vi "vPR_All.vi"(8 "error in (no error)":errorcluster, 9 "結束時間":timestamp=timestamp(3738902301.8455286 s since 1904-01-01), 10 "開始時間":timestamp=timestamp(3738815886.436984 s since 1904-01-01), 11 "DBlink":string="Driver={ODBC Driver 17 for SQL Server};Server=localhost\\SQLEXPRESS;Database=ZDX201;UID=labview;PWD=Dsa@54137926") -> (0 "error out":errorcluster={"status"=TRUE, "code"=-2147217843, "source"="NI_Database_API.lvlib:DB Tools Open Connec (String).vi->WD_assemble_data.vi<ERR>ADO Error: 0x80040E4D\r\nException occured in Microsoft OLE DB Provider for ODBC Drivers: [Microsoft][ODBC Driver 17 for SQL Server][SQL Server]使用者 'labview' 的登入失敗。 in NI_Database_API.lvlib:DB Tools Open Connec (String).vi->WD_assemble_data.vi"}, 3 "Production":T1(array[cluster]))   [LabVIEW 2019]
uses:
  <vilib>/addons/database/Connection.llb/DB Tools Open Connec (String).vi
  <vilib>/addons/database/Connection.llb/Conn Execute.vi
  <vilib>/addons/database/Recordset.llb/Rec Fetch Recordset Data (R).vi
  <vilib>/addons/database/Recordset.llb/Rec Destroy - Connection.vi
  <vilib>/addons/database/_DB Variant To Data/Database Variant To Data.xnode
  <vilib>/addons/database/NI_Database_API.lvlib
panel:
  out "查詢結果":string="SELECT [id]\n      ,[name]\n      ,[barcode A]\n      ,[barcode B]\n      ,[update_time]\n  FROM [ZDX201].[dbo].[workplace_data]\n  where id>0 and id<6\n  order by id"
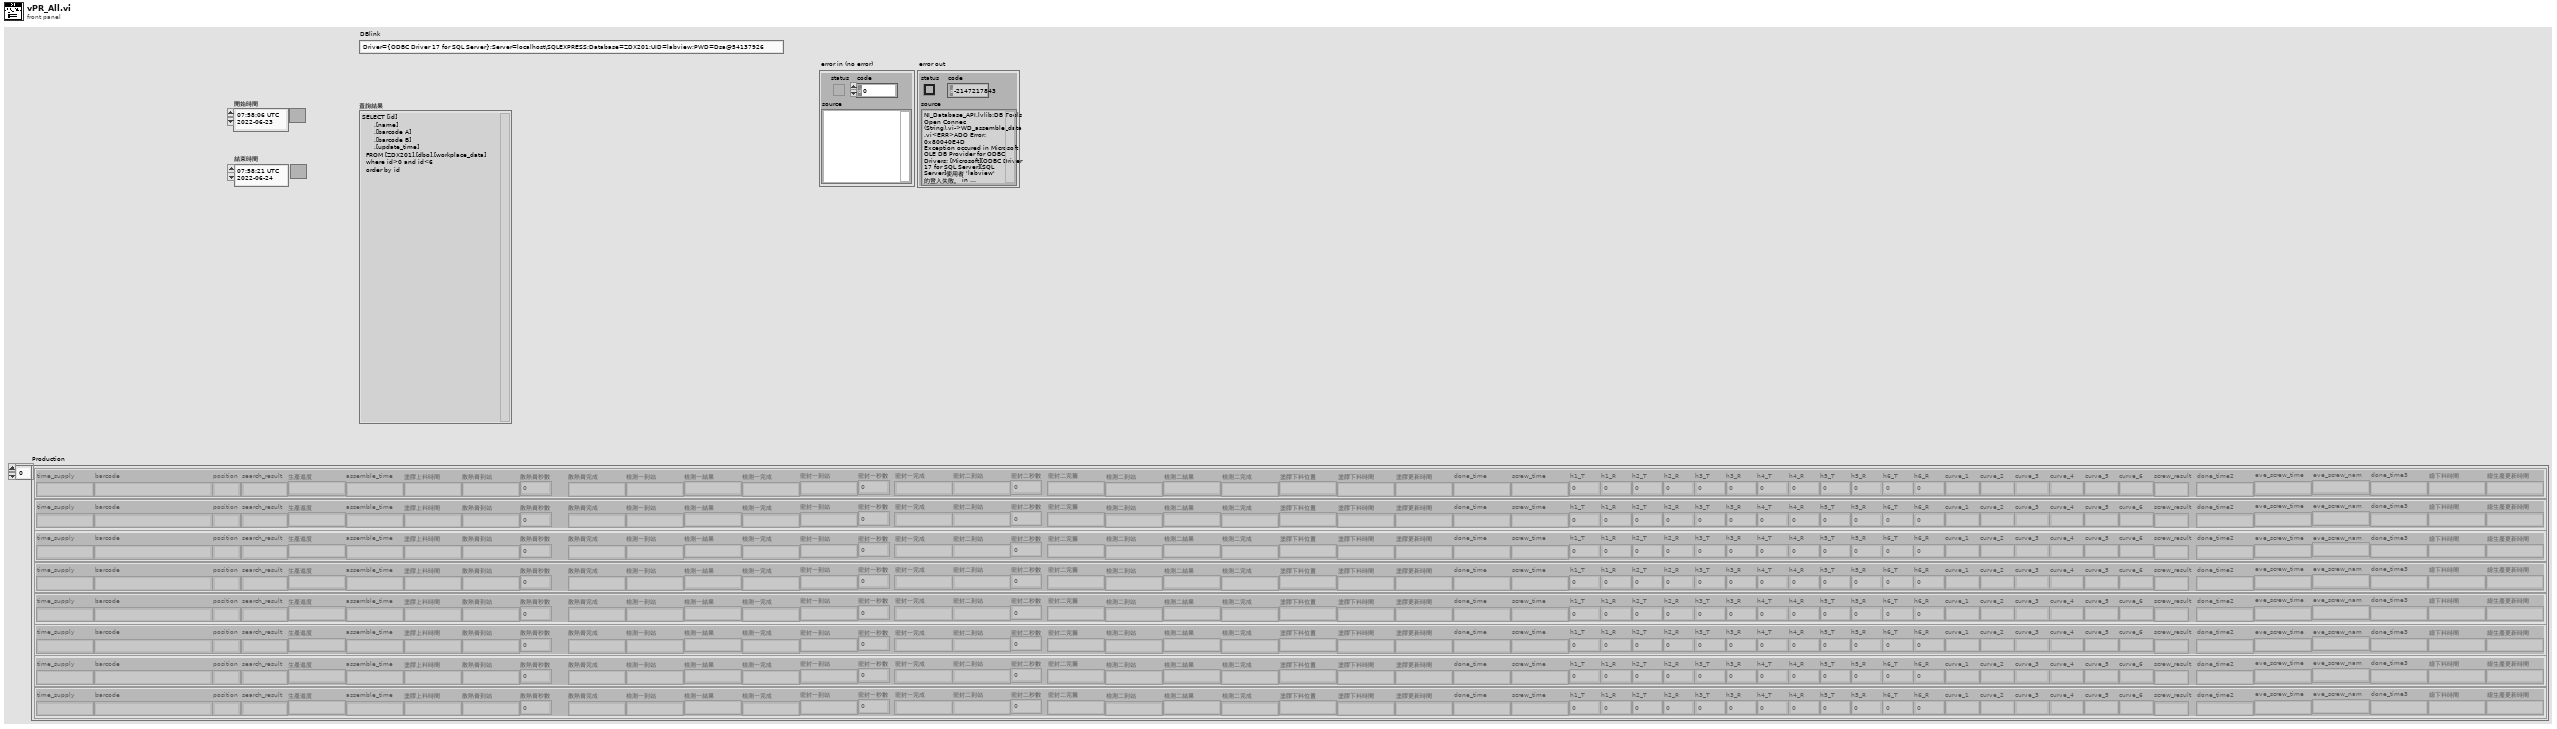
[diagram p1: front panel]
types:
  T1 = cluster{"time_supply":string, "barcode":string, "position":string, "search_result":string, "生產進度":string, "assemble_time":string, "塗膠上料時間":string, "散熱膏到站":string, "散熱膏秒數":dbl, "散熱膏完成":string, "檢測一到站":string, "檢測一結果":string, "檢測一完成":string, "密封一到站":string, "密封一秒數":dbl, "密封一完成":string, "密封二到站":string, "密封二秒數":dbl, "密封二完籌":string, "檢測二到站":string, "檢測二結果":string, "檢測二完成":string, "塗膠下料位置":string, "塗膠下料時間":string, "塗膠更新時間":string, "done_time":string, "screw_time":string, "h1_T":dbl, "h1_R":dbl, "h2_T":dbl, "h2_R":dbl, "h3_T":dbl, "h3_R":dbl, "h4_T":dbl, "h4_R":dbl, "h5_T":dbl, "h5_R":dbl, "h6_T":dbl, "h6_R":dbl, "curve_1":string, "curve_2":string, "curve_3":string, "curve_4":string, "curve_5":string, "curve_6":string, "screw_result":string, "done_time2":string, "eve_screw_time":string, "eve_screw_nam":string, "done_time3":string, "總下料時間":string, "總生產更新時間":string}[]
  T2 = typedef "NI_Database_API.lvlib/Conn ObjectReference.ctl" = refnum<k1>
  T3 = typedef "NI_Database_API.lvlib/Rec ObjectReference.ctl" = refnum<k1>
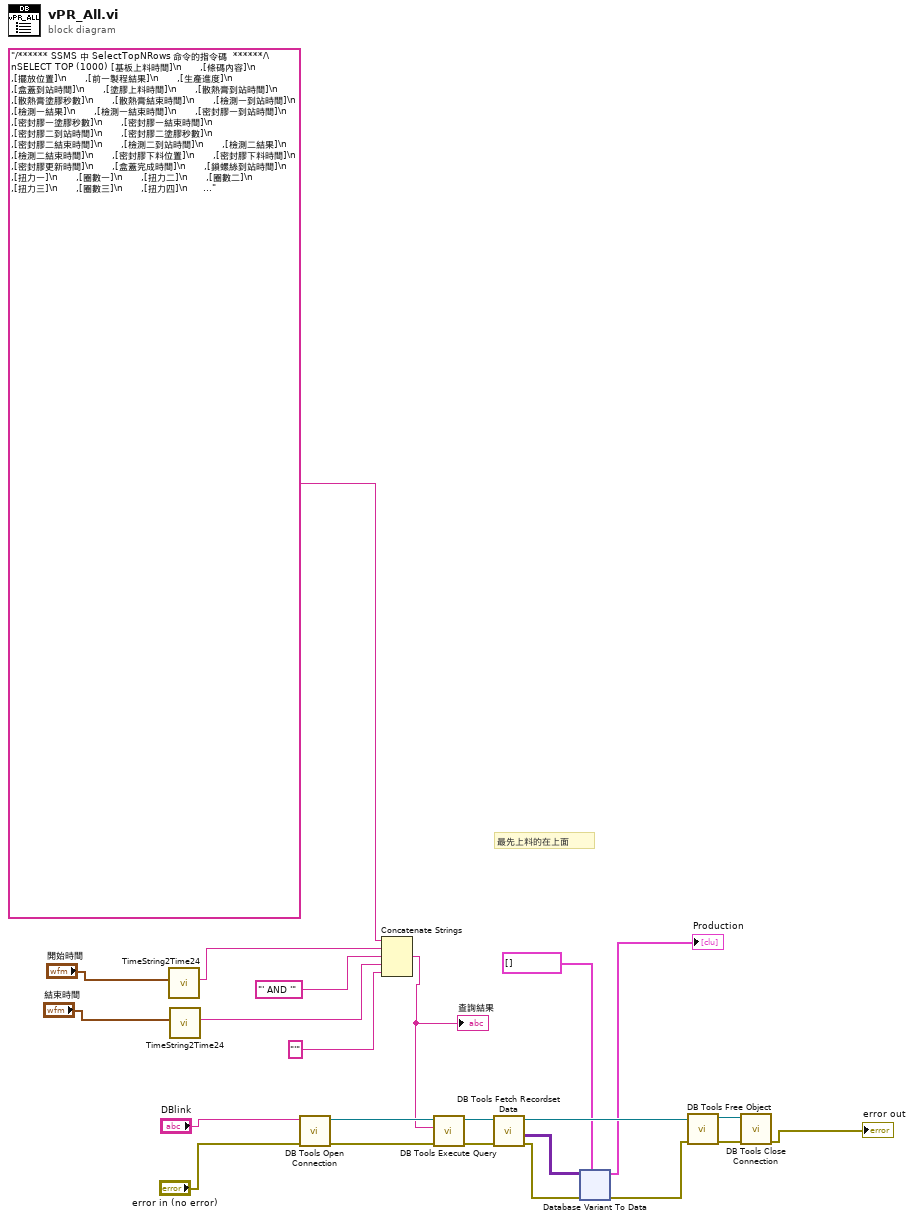
[diagram p0: block diagram]
diagram:
  # "最先上料的在上面"
  n1 = call "TimeString2Time24.vi"("Time Stamp"="開始時間") -> ("時間字串"=w2:string)  [unwired: 9 in, 1 out]
  n2 = call "TimeString2Time24.vi"("Time Stamp"="結束時間") -> ("時間字串"=w1:string)  [unwired: 9 in, 1 out]
  n3 = call-poly <vilib>:"DB Tools Open Connection.vi"("error in (no error)"="error in (no error)", "connection information"="DBlink") -> ("error out"=w23:errorcluster, "connection reference"=w22:T2)  [unwired: 6 in]
  n4 = Concatenate Strings("/****** SSMS 中 SelectTopNRows 命令的指令碼  ******/\nSELECT TOP (1000) [基板上料時間]\n      ,[條碼內容]\n      ,[擺放位置]\n      ,[前一製程結果]\n      ,[生產進度]\n      ,[盒蓋到站時間]\n      ,[塗膠上料時間]\n      ,[散熱膏到站時間]\n      ,[散熱膏塗膠秒數]\n      ,[散熱膏結束時間]\n      ,[檢測一到站時間]\n      ,[檢測一結果]\n      ,[檢測一結束時間]\n      ,[密封膠一到站時間]\n      ,[密封膠一塗膠秒數]\n      ,[密封膠一結束時間]\n      ,[密封膠二到站時間]\n      ,[密封膠二塗膠秒數]\n      ,[密封膠二結束時間]\n      ,[檢測二到站時間]\n      ,[檢測二結果]\n      ,[檢測二結束時間]\n      ,[密封膠下料位置]\n      ,[密封膠下料時間]\n      ,[密封膠更新時間]\n      ,[盒蓋完成時間]\n      ,[鎖螺絲到站時間]\n      ,[扭力一]\n      ,[圈數一]\n      ,[扭力二]\n      ,[圈數二]\n      ,[扭力三]\n      ,[圈數三]\n      ,[扭力四]\n      ,[圈數四]\n      ,[扭力五]\n      ,[圈數五]\n      ,[扭力六]\n      ,[圈數六]\n      ,[曲線檔名一]\n      ,[曲線檔名二]\n      ,[曲線檔名三]\n      ,[曲線檔名四]\n      ,[曲線檔名五]\n      ,[曲線檔名六]\n      ,[鎖固結果]\n      ,[鎖固完成時間]\n      ,[螺絲檢測到站時間]\n      ,[檢測檔名]\n      ,[螺絲檢測完成時間]\n      ,[總下料時間]\n      ,[更新時間]\n  FROM [ZDX201].[dbo].[v_production_glue]\nwhere [總下料時間] between'", w2, "' AND '" ("string"), w1, "'" ("string")) -> (w5:string)
  "查詢結果" <- w5
  n5 = call-poly <vilib>:"DB Tools Execute Query.vi"("error in (no error)"=w23, "SQL query"=w5, "connection reference"=w22) -> ("error out"=w20:errorcluster, "recordset reference"=w21:T3)  [unwired: 5 in]
  n6 = call-poly <vilib>:"DB Tools Fetch Recordset Data.vi"("error in (no error)"=w20, "recordset reference"=w21) -> ("error out"=w15:errorcluster, "recordset data"=w14:variant[][], "recordset reference out"=w16:T3)  [unwired: 3 in]
  n7 = xnode "Database Variant To Data"("database variant"=w14, "error in (no error)"=w15, "type"=T1 [] ("Workplace")) -> ("data"=→"Production":T1, "error out"=w17:errorcluster)
  n8 = call-poly <vilib>:"DB Tools Free Object.vi"("error in (no error)"=w17, "recordset reference"=w16) -> ("error out"=w18:errorcluster, "connection reference"=w19:T2)  [unwired: 8 in]
  n9 = call <vilib>:"DB Tools Close Connection.vi"("error in (no error)"=w18, "connection reference"=w19) -> ("error out"=→"error out":errorcluster)  [unwired: 5 in]
